vi "Pockels Cal-Norm COV.vi"(11 "Coeffecient of variation":dbl) -> (3 "Weighting (rormalised V)":dbl format="%#_6f")   [LabVIEW 2013]
uses:
  <vilib>/gmath/NI_Gmath.lvlib
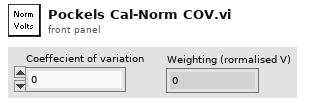
[diagram p1: front panel]
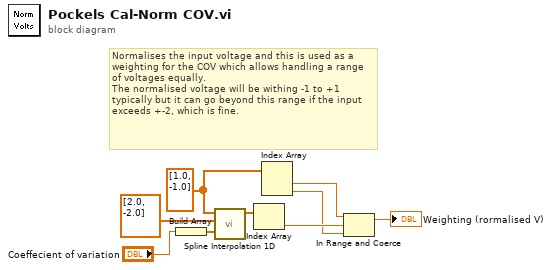
[diagram p0: block diagram]
diagram:
  w3 = dbl[] [1.0, -1.0] ("Y")
  # "Normalises the input voltage and this is used as a weighting for the COV which allows handling a range of voltages equally.\nThe normalised voltage will be withing -1 to +1 typically but it can go beyond this range if the input exceeds +-2, which is fine."
  n1 = Build Array("Coeffecient of variation") -> (w8:dbl[])
  n2 = call <vilib>:"Spline Interpolation 1D.vi"("xi"=w8, "X"=dbl[] [2.0, -2.0] ("Y"), "Y"=w3) -> ("yi"=w6:dbl[])  [unwired: 6 in, 2 out]
  n3 = Index Array(array=w6) -> (element=w5:dbl)  [unwired: 1 in]
  n4 = Index Array(array=w3) -> (element #1=w2:dbl, element #2=w1:dbl)  [unwired: 2 in]
  n5 = In Range and Coerce(upper limit=w2, x=w5, lower limit=w1) -> (coerced(x)=→"Weighting (rormalised V)":dbl)  [unwired: 1 out]
